vi "Cut Motor Power.vi"(10 "f in":dbl, 11 "Sensor Position":dbl) -> (2 "Boolean":bool, 3 "f out":dbl)   [LabVIEW 2018]
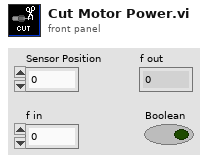
[diagram p1: front panel]
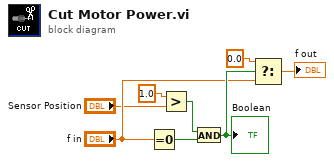
[diagram p0: block diagram]
diagram:
  n1 = Equal To 0?(x="f in") -> (x = 0?=w7:bool)
  n2 = Greater?(x=1.0, y="Sensor Position") -> (0:w6:bool)
  n3 = And(x=w6, y=w7) -> (x .and. y?=w8:bool)
  "Boolean" <- w8
  n4 = Select(t=0.0, s=w8, f="f in") -> (s? t:f=→"f out":dbl)
